vi "Spectrum Configure.vi"(0 "RFmx Handle In":refnum<k21>, 1 "Selector String":string, 5 "RFmx SpecAn Spectrum Configuration":T1={"Span (Hz)"=1000000.0, "Sweep Time Auto"=1, "Sweep Time Interval (s)"=0.001, "RBW Auto"=1, "RBW (Hz)"=10000.0, "RBW Filter Type"=1, "Averaging Enabled"=0, "Averaging Count"=10, "Averaging Type"=0} {"Averaging Type" items=["RMS", "Log", "Scalar", "Max", "Min"]; "Averaging Enabled" items=["False", "True"]; "RBW Auto" items=["False", "True"]; "RBW (Hz)" format="%.3p"; "RBW Filter Type" items=["FFT Based", "Gaussian", "Flat"]; "Sweep Time Auto" items=["False", "True"]; "Sweep Time Interval (s)" format="%.2p"; "Span (Hz)" format="%.3p"}, 11 "error in (no error)":errorcluster) -> (4 "RFmx Handle Out":refnum<k21>, 15 "error out":errorcluster)   [LabVIEW 2016, in "RFmxSpecAn.lvlib"]
uses:
  RFmxSpecAn.lvlib
  <vilib>/RFmx/SpecAn/mx/RFmxSpecAn.llb/RFmxSpecAn Select Measurement (Single).vi
  Typedefs/Spectrum Configuration.ctl
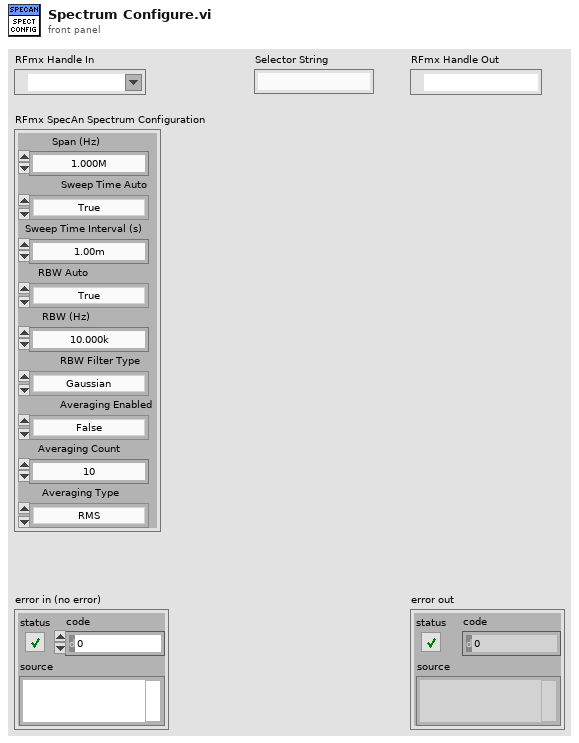
[diagram p1: front panel]
types:
  T1 = typedef "RFmxSpecAn.lvlib/Spectrum Configuration.ctl" = cluster{"Span (Hz)":dbl, "Sweep Time Auto":i32, "Sweep Time Interval (s)":dbl, "RBW Auto":i32, "RBW (Hz)":dbl, "RBW Filter Type":i32, "Averaging Enabled":i32, "Averaging Count":i32, "Averaging Type":i32}
  T2 = enum16{"ACP", "CCDF", "CHP", "FCnt", "Harmonics", "OBW", "SEM", "Spectrum", "Spur", "TXP", "AMPM", "DPD", "IQ", "IM", "NF", "PhaseNoise"}
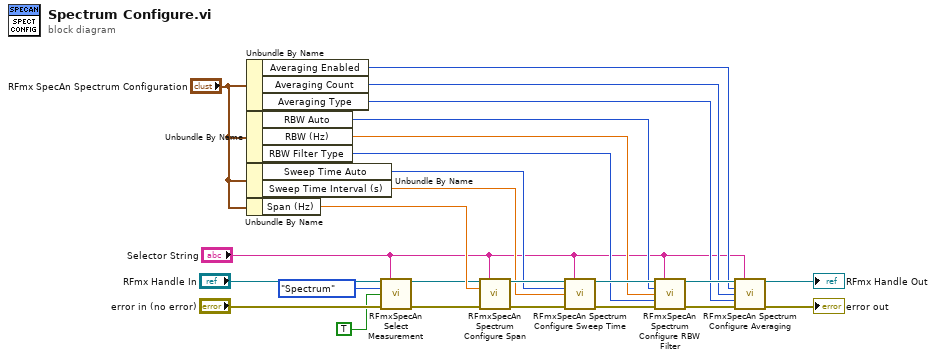
[diagram p0: block diagram]
diagram:
  n1 = Unbundle By Name("RFmx SpecAn Spectrum Configuration") -> ("Averaging Enabled"=w12:i32, "Averaging Count"=w13:i32, "Averaging Type"=w14:i32)
  n2 = Unbundle By Name("RFmx SpecAn Spectrum Configuration") -> ("RBW Auto"=w10:i32, "RBW (Hz)"=w11:dbl, "RBW Filter Type"=w9:i32)
  n3 = Unbundle By Name("RFmx SpecAn Spectrum Configuration") -> ("Sweep Time Auto"=w8:i32, "Sweep Time Interval (s)"=w7:dbl)
  n4 = Unbundle By Name("RFmx SpecAn Spectrum Configuration") -> ("Span (Hz)"=w16:dbl)
  n5 = call-poly <vilib>:"RFmxSpecAn Select Measurement.vi"("Instrument Handle In"="RFmx Handle In", "Selector String"="Selector String", "Measurement"=T2."Spectrum", "Enable All Traces"=TRUE, "error in (no error)"="error in (no error)") -> ("Instrument Handle Out"=w4:refnum<k21>, "error out"=w6:errorcluster)  [unwired: 9 in]
  n6 = call <vilib>:"RFmxSpecAn Spectrum Configure Span.vi"("Instrument Handle In"=w4, "Selector String"="Selector String", "Span (Hz)"=w16, "error in (no error)"=w6) -> ("Instrument Handle Out"=w24:refnum<k21>, "error out"=w23:errorcluster)  [unwired: 10 in]
  n7 = call <vilib>:"RFmxSpecAn Spectrum Configure Sweep Time.vi"("Instrument Handle In"=w24, "Selector String"="Selector String", "Sweep Time Auto"=w8, "Sweep Time Interval (s)"=w7, "error in (no error)"=w23) -> ("Instrument Handle Out"=w22:refnum<k21>, "error out"=w21:errorcluster)  [unwired: 9 in]
  n8 = call <vilib>:"RFmxSpecAn Spectrum Configure RBW Filter.vi"("Instrument Handle In"=w22, "Selector String"="Selector String", "RBW Auto"=w10, "RBW (Hz)"=w11, "RBW Filter Type"=w9, "error in (no error)"=w21) -> ("Instrument Handle Out"=w20:refnum<k21>, "error out"=w19:errorcluster)  [unwired: 8 in]
  n9 = call <vilib>:"RFmxSpecAn Spectrum Configure Averaging.vi"("Instrument Handle In"=w20, "Selector String"="Selector String", "Averaging Enabled"=w12, "Averaging Count"=w13, "Averaging Type"=w14, "error in (no error)"=w19) -> ("Instrument Handle Out"=→"RFmx Handle Out":refnum<k21>, "error out"=→"error out":errorcluster)  [unwired: 8 in]
